vi "Save_Destinations.vi"(8 "error in (no error)":errorcluster, 11 "AB_Build in":refnum<class "AB_Build.lvclass">) -> (0 "error out":errorcluster, 3 "AB_Build out":refnum<class "AB_Build.lvclass">)   [LabVIEW 2020, in "AB_Build.lvclass"]
uses:
  <vilib>/AppBuilder/AB_Classes/Build/AB_Build.lvclass
  <vilib>/AppBuilder/AB_Classes/Build/AB_Build.lvclass/AB_Build.ctl
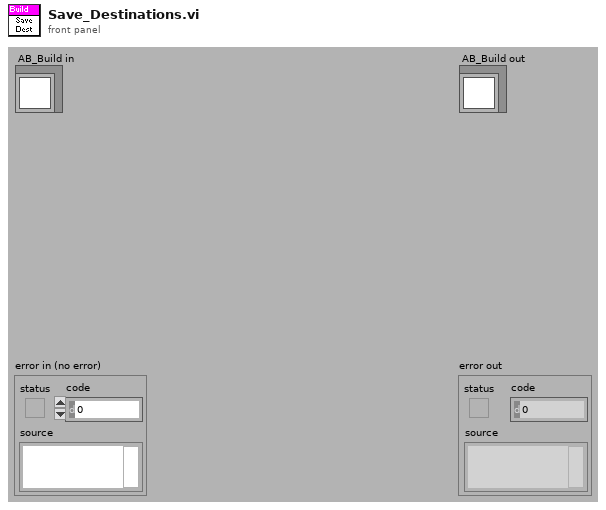
[diagram p1: front panel]
types:
  T1 = typedef "ItemRef.ctl" = u64
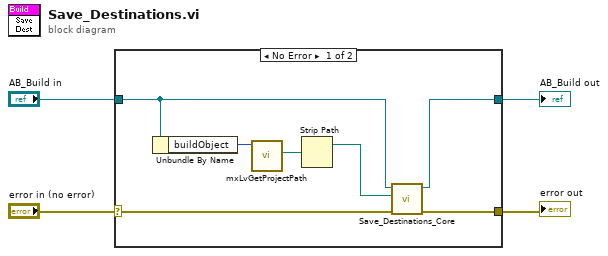
[diagram p0: block diagram]
diagram:
  n1 = case shown="No Error" "error in (no error)" {
    selector: "error in (no error)" -> [w9 w13]
    tunnel: [w8 w13] -> w3
    tunnel: [w10 w12] -> w1
    tunnel: "AB_Build in" -> [w11 w12]
    frame No Error {
      n2 = Unbundle By Name(w11) -> ("buildObject"=w6:T1)
      n3 = call <resource>:"mxLvGetProjectPath.vi"("Item"=w6) -> ("Project Path"=w5:path)  [unwired: 8 in, 2 out]
      n4 = Strip Path(path=w5) -> (stripped path=w7:path)  [unwired: 1 out]
      n5 = call-dynamic "Save_Destinations_Core.vi"("error in (no error)"=w9, "commonPath"=w7, "AB_Build in"=w11) -> ("error out"=w8:errorcluster, "AB_Build out"=w10:refnum<class "AB_Build.lvclass">)  [unwired: 7 in]
    }
    frame Error {
    }
  }
  "error out" <- w3
  "AB_Build out" <- w1
